vi "Get_run_info.vi"(1 "Run Info Cluster In":T1={"Set Point (*C)"=0, "Field (uT)"=0.0, "Soak Time (min)"=30, "Field on/off"=FALSE, "Atmosphere"="1", "Use DB"=enum."DB Yes", "User ID"="", "Batch / Boat ID"="", "User"="", "Note"="", "Field on (C)"=0.0, "Field off (C)"=0.0, "email address"="", "Control ramp"=FALSE, "Ramp rate"=1.0, "Contact Me"=enum."No Selection", "Test e-mail"=FALSE, "Cellular Provider"=""} {"Ramp rate" min=1.0 max=100.0}) -> (0 "Run Info Cluster Out":T1={"Set Point (*C)"=0, "Field (uT)"=0.0, "Soak Time (min)"=30, "Field on/off"=FALSE, "Atmosphere"="1", "Use DB"=enum."DB Yes", "User ID"="", "Batch / Boat ID"="", "User"="", "Note"="", "Field on (C)"=0.0, "Field off (C)"=0.0, "email address"="", "Control ramp"=FALSE, "Ramp rate"=0.0, "Contact Me"=enum."E-mail", "Test e-mail"=FALSE, "Cellular Provider"=""})   [LabVIEW 2009]
doc: "Displays window to gather information about user and run conditions.\nOutput is bundled cluster with:\n1) Use DB boolean\n2) DB User ID\n3) non-DB User Name\n4) Field on/off boolean\n5) Field magnitude\n6) Set point\n7) Soak time\n8) Atmosphere flag\n9) Note"
panel:
  in  "Abort":bool
  in  "Continue":bool
  # "Run Information"
  # "(deg/min)"
  # "User Information"
  # "Run Information"
  # "(deg/min)"
  # "E-mail or text me when done at:"
  # "(enter e-mail address or phone number)"
  # "User Information"
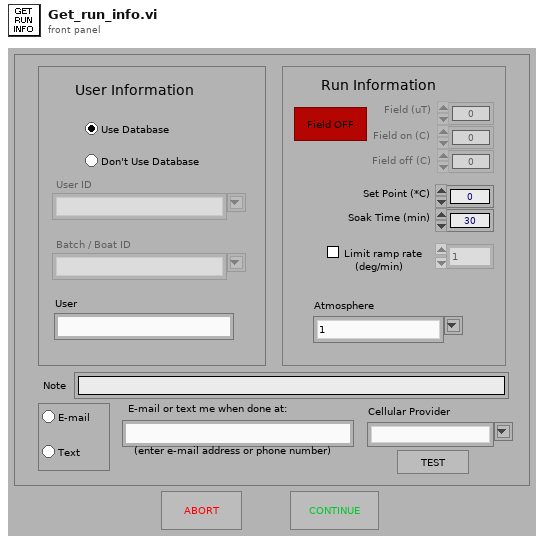
[diagram p1: front panel]
types:
  T1 = cluster{"Set Point (*C)":u32, "Field (uT)":dbl, "Soak Time (min)":u32, "Field on/off":bool, "Atmosphere":string, "Use DB":enum32{"DB Yes", "DB no"}, "User ID":string, "Batch / Boat ID":string, "User":string, "Note":string, "Field on (C)":dbl, "Field off (C)":dbl, "email address":string, "Control ramp":bool, "Ramp rate":dbl, "Contact Me":enum32{"No Selection", "E-mail", "Text"}, "Test e-mail":bool, "Cellular Provider":string}
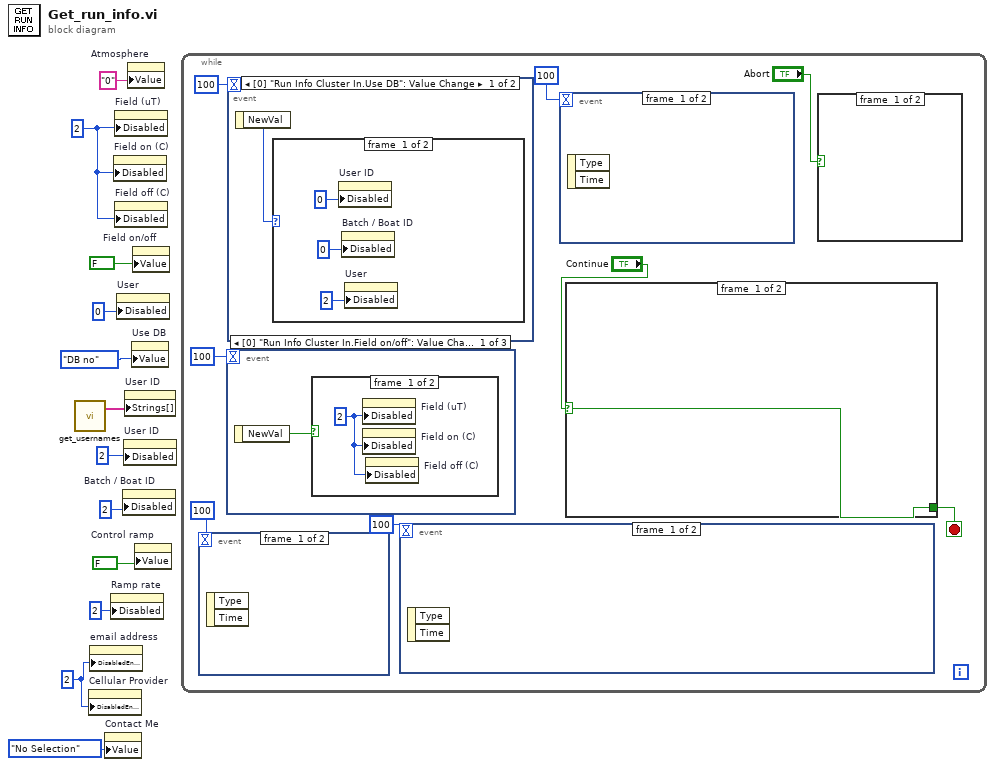
[diagram p0: block diagram]
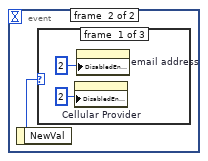
[diagram p2: hidden frame]
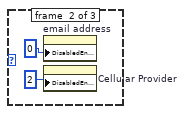
[diagram p3: hidden frame]
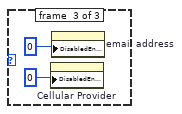
[diagram p4: hidden frame]
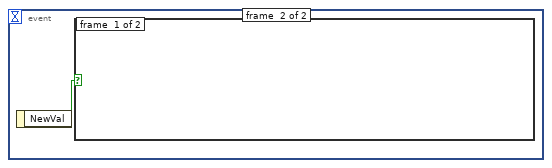
[diagram p5: hidden frame]
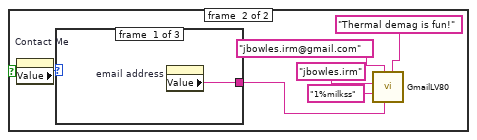
[diagram p6: hidden frame]
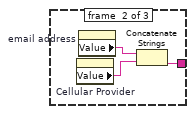
[diagram p7: hidden frame]
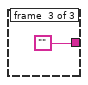
[diagram p8: hidden frame]
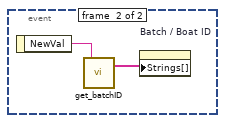
[diagram p9: hidden frame]
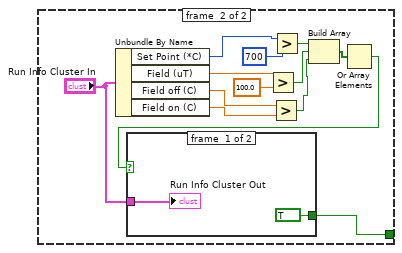
[diagram p10: hidden frame]
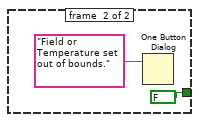
[diagram p11: hidden frame]
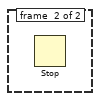
[diagram p12: hidden frame]
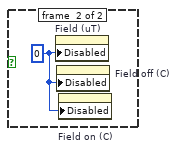
[diagram p13: hidden frame]
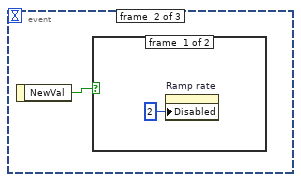
[diagram p14: hidden frame]
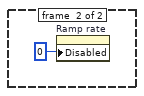
[diagram p15: hidden frame]
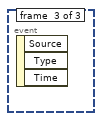
[diagram p16: hidden frame]
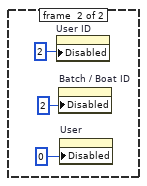
[diagram p17: hidden frame]
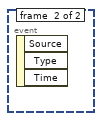
[diagram p18: hidden frame]
diagram:
  w2 = u8 2 ("Disabled")
  w5 = u8 2 ("Disabled")
  n1 = call "get_usernames.vi"() -> ("UserID output"=w12:string[])  [unwired: 1 in, 2 out]
  n2 = property on="Cellular Provider" class="CmbBox"("DisabledEnum"=w2) -> ()  [unwired: 2 in, 2 out]
  n3 = property on="email address" class="Str"("DisabledEnum"=w2) -> ()  [unwired: 2 in, 2 out]
  n4 = property on="Contact Me" class="RadioBtnsControl (strict)"("Value"=enum32{"No Selection", "E-mail", "Text"}."No Selection") -> ()  [unwired: 2 in, 2 out]
  n5 = property on="Ramp rate" class="DigNum (strict)"("Disabled"=u8 2) -> ()  [unwired: 2 in, 2 out]
  n6 = property on="Field on (C)" class="DigNum (strict)"("Disabled"=w5) -> ()  [unwired: 2 in, 2 out]
  n7 = property on="Field (uT)" class="DigNum (strict)"("Disabled"=w5) -> ()  [unwired: 2 in, 2 out]
  n8 = property on="Field off (C)" class="DigNum (strict)"("Disabled"=w5) -> ()  [unwired: 2 in, 2 out]
  n9 = property on="User" class="Str"("Disabled"=u8 0) -> ()  [unwired: 2 in, 2 out]
  n10 = property on="Batch / Boat ID" class="CmbBox"("Disabled"=u8 2) -> ()  [unwired: 2 in, 2 out]
  n11 = property on="User ID" class="CmbBox"("Disabled"=u8 2) -> ()  [unwired: 2 in, 2 out]
  n12 = property on="User ID" class="CmbBox"("Strings[]"=w12) -> ()  [unwired: 2 in, 2 out]
  n13 = property on="Atmosphere" class="CmbBox"("Value"="0") -> ()  [unwired: 2 in, 2 out]
  n14 = property on="Use DB" class="RadioBtnsControl (strict)"("Value"=enum32{"DB Yes", "DB no"}."DB no" ("Use DB")) -> ()  [unwired: 2 in, 2 out]
  n15 = property on="Field on/off" class="Bool (strict)"("Value"=FALSE) -> ()  [unwired: 2 in, 2 out]
  n16 = property on="Control ramp" class="Bool (strict)"("Value"=FALSE) -> ()  [unwired: 2 in, 2 out]
  n17 = while {
    stop <- w18 stop-if-true
    n18 = event shown="[1] \"Run Info Cluster In.Contact Me\": Value Change" {
      selector: _ -> [_ _]
      dyn-events: _ -> [_ _]
      timeout: 100 -> [_ _]
      event #0 {
        n19 = event-data() -> ()  [unwired: 1 in, 2 out]
      }
      event #1 {
        n20 = event-data() -> ("NewVal"=w21:enum32{"No Selection", "E-mail", "Text"})  [unwired: 1 in]
        n21 = case shown="\"No Selection\", Default" w21 {
          frame #0 {
            n22 = property on="Cellular Provider" class="CmbBox"("DisabledEnum"=u8 2 ("Disabled")) -> ()  [unwired: 2 in, 2 out]
            n23 = property on="email address" class="Str"("DisabledEnum"=u8 2 ("Disabled")) -> ()  [unwired: 2 in, 2 out]
          }
          frame #1 {
            n24 = property on="email address" class="Str"("DisabledEnum"=u8 0 ("Disabled")) -> ()  [unwired: 2 in, 2 out]
            n25 = property on="Cellular Provider" class="CmbBox"("DisabledEnum"=u8 2 ("Disabled")) -> ()  [unwired: 2 in, 2 out]
          }
          frame #2 {
            n26 = property on="Cellular Provider" class="CmbBox"("DisabledEnum"=u8 0 ("Disabled")) -> ()  [unwired: 2 in, 2 out]
            n27 = property on="email address" class="Str"("DisabledEnum"=u8 0 ("Disabled")) -> ()  [unwired: 2 in, 2 out]
          }
        }
      }
    }
    n28 = event shown="[0] \"Run Info Cluster In.Field on/off\": Value Change" {
      selector: _ -> [_ _ _]
      dyn-events: _ -> [_ _ _]
      timeout: 100 -> [_ _ _]
      event #0 {
        n29 = event-data() -> ("NewVal"=w60:bool)  [unwired: 1 out]
        n30 = case shown="False" w60 {
          frame #0 {
            w61 = u8 2 ("Disabled")
            n31 = property on="Field (uT)" class="DigNum (strict)"("Disabled"=w61) -> ()  [unwired: 2 in, 2 out]
            n32 = property on="Field on (C)" class="DigNum (strict)"("Disabled"=w61) -> ()  [unwired: 2 in, 2 out]
            n33 = property on="Field off (C)" class="DigNum (strict)"("Disabled"=w61) -> ()  [unwired: 2 in, 2 out]
          }
          frame #1 {
            w62 = u8 0 ("Disabled")
            n34 = property on="Field (uT)" class="DigNum (strict)"("Disabled"=w62) -> ()  [unwired: 2 in, 2 out]
            n35 = property on="Field off (C)" class="DigNum (strict)"("Disabled"=w62) -> ()  [unwired: 2 in, 2 out]
            n36 = property on="Field on (C)" class="DigNum (strict)"("Disabled"=w62) -> ()  [unwired: 2 in, 2 out]
          }
        }
      }
      event #1 {
        n37 = event-data() -> ("NewVal"=w63:bool)  [unwired: 1 out]
        n38 = case shown="False" w63 {
          frame #0 {
            n39 = property on="Ramp rate" class="DigNum (strict)"("Disabled"=u8 2) -> ()  [unwired: 2 in, 2 out]
          }
          frame #1 {
            n40 = property on="Ramp rate" class="DigNum (strict)"("Disabled"=u8 0) -> ()  [unwired: 2 in, 2 out]
          }
        }
      }
      event #2 {
        n41 = event-data() -> ()  [unwired: 4 out]
      }
    }
    n42 = event shown="[0] \"Run Info Cluster In.Use DB\": Value Change" {
      selector: _ -> [_ _]
      dyn-events: _ -> [_ _]
      timeout: 100 -> [_ _]
      event #0 {
        n43 = event-data() -> ("NewVal"=w66:enum32{"DB Yes", "DB no"})  [unwired: 1 out]
        n44 = case shown="\"DB no\"" w66 {
          frame #0 {
            n45 = property on="User ID" class="CmbBox"("Disabled"=u8 0) -> ()  [unwired: 2 in, 2 out]
            n46 = property on="Batch / Boat ID" class="CmbBox"("Disabled"=u8 0) -> ()  [unwired: 2 in, 2 out]
            n47 = property on="User" class="Str"("Disabled"=u8 2) -> ()  [unwired: 2 in, 2 out]
          }
          frame #1 {
            n48 = property on="User ID" class="CmbBox"("Disabled"=u8 2) -> ()  [unwired: 2 in, 2 out]
            n49 = property on="Batch / Boat ID" class="CmbBox"("Disabled"=u8 2) -> ()  [unwired: 2 in, 2 out]
            n50 = property on="User" class="Str"("Disabled"=u8 0) -> ()  [unwired: 2 in, 2 out]
          }
        }
      }
      event #1 {
        n51 = event-data() -> ()  [unwired: 4 out]
      }
    }
    n52 = event shown="[1] \"Run Info Cluster In.Test e-mail\": Value Change" {
      selector: _ -> [_ _]
      dyn-events: _ -> [_ _]
      timeout: 100 -> [_ _]
      event #0 {
        n53 = event-data() -> ()  [unwired: 1 in, 2 out]
      }
      event #1 {
        n54 = event-data() -> ("NewVal"=w28:bool)  [unwired: 1 in]
        n55 = case shown="True" w28 {
          frame #0 {
          }
          frame #1 {
            n56 = property on="Contact Me" class="RadioBtnsControl (strict)"() -> ("Value"=w34:enum32{"No Selection", "E-mail", "Text"})  [unwired: 2 in, 2 out]
            n57 = case shown="\"Text\"" w34 {
              tunnel: [w35 w36 ""] -> w29
              frame #0 {
                n58 = property on="email address" class="Str"() -> ("Value"=w35:string)  [unwired: 2 in, 2 out]
              }
              frame #1 {
                n59 = property on="Cellular Provider" class="CmbBox"() -> ("Value"=w37:string)  [unwired: 2 in, 2 out]
                n60 = property on="email address" class="Str"() -> ("Value"=w38:string)  [unwired: 2 in, 2 out]
                n61 = Concatenate Strings(w38, w37) -> (w36:string)
              }
              frame #2 {
              }
            }
            n62 = call "GmailLV80.vi"("Subject"="Thermal demag is fun!", "Recipient's Email Address"=w29, "Sender's Email Address (eg: LabVIEW@gmail.com)"="jbowles.irm@gmail.com", "GMAIL Account Password"="1%milkss", "GMAIL Account User ID"="jbowles.irm") -> ()  [unwired: 3 in, 4 out]
          }
        }
      }
    }
    n63 = event shown="[1] \"Run Info Cluster In.User ID\": Value Change" {
      selector: _ -> [_ _]
      dyn-events: _ -> [_ _]
      timeout: 100 -> [_ _]
      event #0 {
        n64 = event-data() -> ()  [unwired: 3 out]
      }
      event #1 {
        n65 = event-data() -> ("NewVal"=w40:string)  [unwired: 1 out]
        n66 = call "get_batchID.vi"("UserID"=w40) -> ("BatchID output"=w41:string[])  [unwired: 1 in, 1 out]
        n67 = property on="Batch / Boat ID" class="CmbBox"("Strings[]"=w41) -> ()  [unwired: 2 in, 2 out]
      }
    }
    n68 = case shown="True" "Continue" {
      selector: "Continue" -> [w42 _]
      tunnel: [w42 w51] -> w18
      frame #0 {
      }
      frame #1 {
        n69 = Unbundle By Name("Run Info Cluster In") -> ("Set Point (*C)"=w53:u32, "Field (uT)"=w52:dbl, "Field off (C)"=w48:dbl, "Field on (C)"=w47:dbl)
        n70 = Greater?(x=w52, y=100.0) -> (0:w46:bool)
        n71 = Greater?(x=w48, y=w47) -> (0:w45:bool)
        n72 = Greater?(x=w53, y=u32 700) -> (0:w49:bool)
        n73 = Build Array(w49, w46, w45) -> (w44:bool[])
        n74 = Or Array Elements(Boolean array=w44) -> (logical OR=w43:bool)
        n75 = case shown="False" w43 {
          tunnel: [TRUE FALSE] -> w51
          tunnel: "Run Info Cluster In" -> [w56 _]
          frame #0 {
            "Run Info Cluster Out" <- w56
          }
          frame #1 {
            n76 = One Button Dialog(message="Field or Temperature set out of bounds.") -> ()  [unwired: 2 out]
          }
        }
      }
    }
    n77 = case shown="False" "Abort" {
      frame #0 {
      }
      frame #1 {
        n78 = Stop() -> ()  [unwired: 1 out]
      }
    }
  }
